vi "TSM SSC DAQmx Read TEDS.vi"(0 "TSM DAQmx In":T2, 11 "error in (no error)":errorcluster) -> (4 "TSM DAQmx Out":T2, 6 "SSC TEDS BitStream":T1[][](array[typedef]), 15 "error out":errorcluster)   [LabVIEW 2020]
doc: "Reads the TEDS bitstream in the order of SSC."
uses:
  Pin Map/TSM DAQmx Multi-Task.ctl
  <vilib>/NI_TestStand_SemiconductorModule/NI_TestStand_Semiconductor_Module.lvlibp/PinMap/PinQueryContext/MultiplePinMultipleSessionQueryContext/MultiplePinMultipleSessionQueryContext.lvclass
  Pin Map/SSC DAQmx.ctl
  SSC DAQmx/Typedefs/SSC TEDS Bitstream.ctl
  da5b0c48-7a5c-4428-9fc9-c6a8fda1cc90.vi
  Shared SubVIs/Channel List to Pins.vi
  Shared SubVIs/Trim Whitespace [Inlined].vi
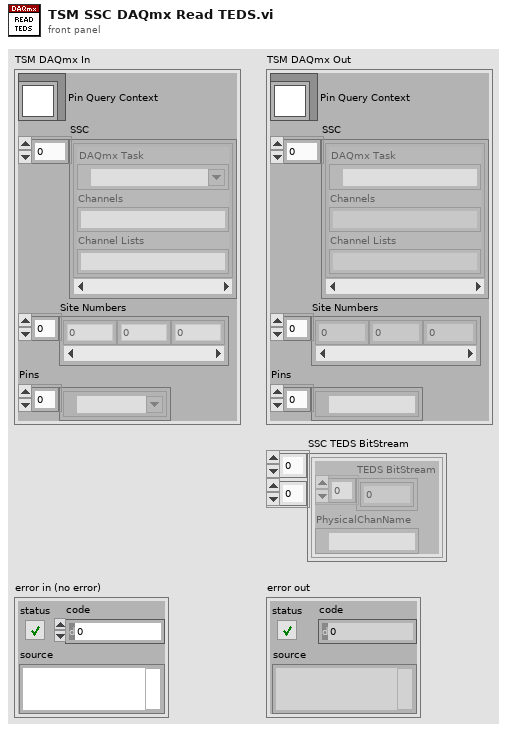
[diagram p1: front panel]
types:
  T1 = typedef "SSC TEDS Bitstream.ctl" = cluster{"TEDS BitStream":u8[], "PhysicalChanName":tag}
  T2 = typedef "TSM DAQmx Multi-Task.ctl" = cluster{"Pin Query Context":refnum<class "MultiplePinMultipleSessionQueryContext.lvclass">, "SSC":T3[], "Site Numbers":i32[], "Pins":tag[]}
  T3 = typedef "SSC DAQmx.ctl" = cluster{"DAQmx Task ":refnum<k21>, "Channels":string, "Channel Lists":string}
  T4 = typedef "Digital 2D Location Array in a Cluster.ctl" = cluster{"Digital 2D Location Array":T5[]}
  T5 = typedef "Digital 2D Location.ctl" = cluster{"Row":i32, "Col":i32}
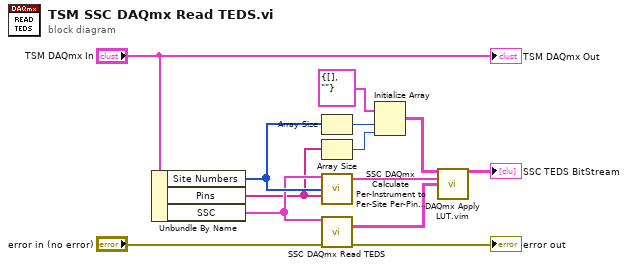
[diagram p0: block diagram]
diagram:
  n1 = Unbundle By Name("TSM DAQmx In") -> ("Site Numbers"=w8:i32[], "Pins"=w1:tag[], "SSC"=w6:T3[])
  n2 = Array Size(array=w8) -> (size(s)=w9:i32)
  n3 = Array Size(array=w1) -> (size(s)=w10:i32)
  n4 = call "SSC DAQmx Calculate Per-Instrument to Per-Site Per-Pin LUT.vi"("DAQmx SSC in"=w6, "Sites"=w8, "Pins"=w1) -> ("Per-Task to Per-Site Per-Pin LUT"=w4:T4[])  [unwired: 12 in]
  n5 = call "SSC DAQmx Read TEDS.vi"("DAQmx SSC in"=w6, "error in"="error in (no error)") -> ("SSC TEDS BitStream"=w5:T1[][], "error out"=→"error out":errorcluster)  [unwired: 11 in, 1 out]
  n6 = Initialize Array(T1 {"TEDS BitStream"=[], "PhysicalChanName"=""}, w9, w10) -> (w11:T1[][])
  n7 = call "DAQmx Apply LUT.vim"("Initialized Array"=w11, "LUT"=w4, "Results to Apply LUT to"=w5) -> ("Array Out"=→"SSC TEDS BitStream":T1[][])  [unwired: 12 in]
  "TSM DAQmx Out" <- "TSM DAQmx In"
